vi "Búsqueda_Receta.vi"(10 "Receta":T2 {"Recetas LS Electric"."Modbus LS-Electric"."Delay respuesta" min=1 max=250 format="%.0f mseg."; "Recetas LS Electric"."Modbus LS-Electric"."Formato RS485" items=["RTU 8-N-1", "RTU 8-N-2", "RTU 8-E-1", "RTU 8-O-1"]; "Recetas LS Electric"."Modbus LS-Electric"."Velocidad datos" items=["1200 bps", "2400 bps", "4800 bps", "9600 bps", "19200 bps", "38400 bps", "56 kbps", "115 kbps"]; "Recetas LS Electric"."Modbus LS-Electric"."Identificador" min=1 max=250; "Recetas LS Electric"."Motor LS-Electric"."Voltaje nominal" min=170 max=480 format="%.0f V"; "Recetas LS Electric"."Motor LS-Electric"."Potencia nominal" items=["0.2 kW", "0.4 kW", "0.75 kW", "1.1 kW", "1.5 kW", "2.2 kW", "3.0 kW", "3.7 kW", "4.0 kW", "5.5 kW", "7.5 kW", "11.kW"]; "Recetas LS Electric"."Motor LS-Electric"."T. Desaceleración" format="%#_g seg"; "Recetas LS Electric"."Motor LS-Electric"."T. Aceleración" format="%#_g seg"; "Recetas LS Electric"."Motor LS-Electric"."Frecuencia máxima" format="%#_g Hz"; "Recetas LS Electric"."Motor LS-Electric"."Frecuencia mínima" format="%#_g Hz"; "Recetas LS Electric"."Motor LS-Electric"."Polos" min=2 max=48; "Recetas LS Electric"."Motor LS-Electric"."Velocidad nominal" format="%.0f rpm"; "Recetas LS Electric"."Motor LS-Electric"."Corriente nominal" format="%#_g Amp"; "Recetas LS Electric"."Motor LS-Electric"."Corriente sin carga" format="%#_g Amp"; "Recetas LS Electric"."Motor LS-Electric"."Frecuencia nominal" items=["60 Hz", "50 Hz"]; "Recetas LS Electric"."Referencias LS-Electric"."Referencia velocidad 2" items=["No asignar"=0, "Analógica (AI1)"=1, "Analógica (AI2)"=2, "Analógica (AI3)"=3, "Modbus"=164, "Potenciómetro (AIU1)"=183]; "Recetas LS Electric"."Referencias LS-Electric"."Referencia arranque 2" items=["Terminales"=1, "Modbus"=10]; "Recetas LS Electric"."Referencias LS-Electric"."Referencia velocidad 1" items=["No asignar"=0, "Analógica (AI1)"=1, "Analógica (AI2)"=2, "Analógica (AI3)"=3, "Modbus"=164, "Potenciómetro (AIU1)"=183]; "Recetas LS Electric"."Referencias LS-Electric"."Referencia arranque 1" items=["Terminales"=1, "Modbus"=10]; "Recetas LS Electric"."I/O LS-Electric"."Relevador 2" items=["Modbus"=0, "FDT-1"=1, "FDT-2"=2, "FDT-3"=3, "FDT-4"=4, "Sobrecarga"=5, "Sobrevoltaje"=10, "Bajo voltaje"=11, "Sobrecalentamiento"=12, "RUN"=14, "STOP"=15, "Listo"=22]; "Recetas LS Electric"."I/O LS-Electric"."Relevador 1" items=["Modbus"=0, "FDT-1"=1, "FDT-2"=2, "FDT-3"=3, "FDT-4"=4, "Sobrecarga"=5, "Sobrevoltaje"=10, "Bajo voltaje"=11, "Sobrecalentamiento"=12, "RUN"=14, "STOP"=15, "Listo"=22]; "Recetas LS Electric"."I/O LS-Electric"."Entrada 5 (P5)" items=["No asignar"=0, "FWD"=1, "REV"=2, "Reset"=3, "Fallo auxiliar (BX)"=5, "Habilitar RUN"=13, "3 hilos"=14, "Segunda referencia"=15, "Segundo motor"=26]; "Recetas LS Electric"."I/O LS-Electric"."Entrada 4 (P4)" items=["Sin asignar"=0, "FWD"=1, "REV"=2, "Reset"=3, "Fallo auxiliar (BX)"=5, "Habilitar RUN"=13, "3 hilos"=14, "Segunda referencia"=15, "Segundo motor"=26]; "Recetas LS Electric"."I/O LS-Electric"."Entrada 3 (P3)" items=["No asignar"=0, "FWD"=1, "REV"=2, "Reset"=3, "Fallo auxiliar (BX)"=5, "Habilitar RUN"=13, "3 hilos"=14, "Segunda referencia"=15, "Segundo motor"=26]; "Recetas LS Electric"."I/O LS-Electric"."Entrada 2 (P2)" items=["No asignar"=0, "FWD"=1, "REV"=2, "Reset"=3, "Fallo auxiliar (BX)"=5, "Habilitar RUN"=13, "3 hilos"=14, "Segunda referencia"=15, "Segundo motor"=26]; "Recetas LS Electric"."I/O LS-Electric"."Entrada 1 (P1)" items=["No asignar"=0, "FWD"=1, "REV"=2, "Reset"=3, "Fallo auxiliar (BX)"=5, "Habilitar RUN"=13, "3 hilos"=14, "Segunda referencia"=15, "Segundo motor"=26]; "Recetas ABB"."Referencias ABB"."Referencia velocidad 2" items=["No asignar"=0, "Analógica (AI1)"=1, "Analógica (AI2)"=2, "Analógica (AI3)"=3, "Modbus"=164, "Potenciómetro (AIU1)"=183]; "Recetas ABB"."Referencias ABB"."Referencia arranque 2" items=["Terminales"=1, "Modbus"=10]; "Recetas ABB"."Referencias ABB"."Referencia velocidad 1" items=["No asignar"=0, "Analógica (AI1)"=1, "Analógica (AI2)"=2, "Analógica (AI3)"=3, "Modbus"=164, "Potenciómetro (AIU1)"=183]; "Recetas ABB"."Referencias ABB"."Referencia arranque 1" items=["Terminales"=1, "Modbus"=10]; "Recetas ABB"."I/O ABB"."Entrada 4 (DI4)" items=["Sin asignar"=0, "Referencia vel. 2"=1, "Referencia vel. 3"=2, "Fallo auxiliar"=12, "Reset"=13, "Entrada lógica 1"=24, "Entrada lógica 2"=25]; "Recetas ABB"."I/O ABB"."Entrada 3 (DI3)" items=["No asignar"=0, "Referencia vel. 2"=1, "Referencia vel. 3"=2, "Fallo auxiliar"=12, "Reset"=13, "Entrada lógica 1"=24, "Entrada lógica 2"=25]; "Recetas ABB"."I/O ABB"."Entrada 2 (DI2)" items=["No asignar"=0, "Referencia vel. 2"=1, "Referencia vel. 3"=2, "Fallo auxiliar"=12, "Reset"=13, "Entrada lógica 1"=24, "Entrada lógica 2"=25, "REV 2 hilos"=50, "DIR 3 hilos"=51]; "Recetas ABB"."I/O ABB"."Entrada 1 (DI1)" items=["No asignar"=0, "Referencia vel. 2"=1, "Referencia vel. 3"=2, "Fallo auxiliar"=12, "Reset"=13, "Entrada lógica 1"=24, "Entrada lógica 2"=25, "FWD 2 hilos"=48, "RUN 3 hilos"=49]; "Recetas Delta"."Referencias Delta"."Referencia velocidad 2" items=["No asignar"=0, "Analógica (AI1)"=1, "Analógica (AI2)"=2, "Analógica (AI3)"=3, "Modbus"=164, "Potenciómetro (AIU1)"=183]; "Recetas Delta"."Referencias Delta"."Referencia arranque 2" items=["Terminales"=1, "Modbus"=10]; "Recetas Delta"."Referencias Delta"."Referencia velocidad 1" items=["No asignar"=0, "Analógica (AI1)"=1, "Analógica (AI2)"=2, "Analógica (AI3)"=3, "Modbus"=164, "Potenciómetro (AIU1)"=183]; "Recetas Delta"."Referencias Delta"."Referencia arranque 1" items=["Terminales"=1, "Modbus"=10]; "Recetas Delta"."I/O Delta"."Entrada 6 (MI6)" items=["Listo/Fallo"=0, "A frecuencia"=1, "Alimentación"=2, "Sobrefrecuencia"=6, "Sobrecorriente"=7, "Sobretensión"=8, "Modbus"=13]; "Recetas Delta"."I/O Delta"."Entrada 5 (MI5)" items=["Listo/Fallo"=0, "A frecuencia"=1, "Alimentación"=2, "Sobrefrecuencia"=6, "Sobrecorriente"=7, "Sobretensión"=8, "Modbus"=13]; "Recetas Delta"."I/O Delta"."Entrada 4 (MI4)" items=["Sin asignar"=0, "Referencia vel. 2"=1, "Referencia vel. 3"=2, "Fallo auxiliar"=12, "Reset"=13, "Entrada lógica 1"=24, "Entrada lógica 2"=25]; "Recetas Delta"."I/O Delta"."Entrada 3 (MI3)" items=["No asignar"=0, "Referencia vel. 2"=1, "Referencia vel. 3"=2, "Fallo auxiliar"=12, "Reset"=13, "Entrada lógica 1"=24, "Entrada lógica 2"=25]; "Recetas Delta"."I/O Delta"."Entrada 2 (MI2)" items=["No asignar"=0, "Referencia vel. 2"=1, "Referencia vel. 3"=2, "Fallo auxiliar"=12, "Reset"=13, "Entrada lógica 1"=24, "Entrada lógica 2"=25, "REV 2 hilos"=50, "DIR 3 hilos"=51]; "Recetas Delta"."I/O Delta"."Entrada 1 (MI1)" items=["No asignar"=0, "Referencia vel. 2"=1, "Referencia vel. 3"=2, "Fallo auxiliar"=12, "Reset"=13, "Entrada lógica 1"=24, "Entrada lógica 2"=25, "FWD 2 hilos"=48, "RUN 3 hilos"=49]; "Recetas Schneider"."I/O Schneider"."Transistor" items=["Listo/Fallo"=0, "A frecuencia"=1, "Alimentación"=2, "Sobrefrecuencia"=6, "Sobrecorriente"=7, "Sobretensión"=8, "Modbus"=13]; "Recetas Schneider"."I/O Schneider"."Relevador 2 (R2)" items=["Listo/Fallo"=0, "A frecuencia"=1, "Alimentación"=2, "Sobrefrecuencia"=6, "Sobrecorriente"=7, "Sobretensión"=8, "Modbus"=13]; "Recetas Schneider"."I/O Schneider"."Relevador 1 (R1)" items=["Listo/Fallo"=0, "A frecuencia"=1, "Alimentación"=2, "Sobrefrecuencia"=6, "Sobrecorriente"=7, "Sobretensión"=8, "Modbus"=13]; "Recetas Schneider"."I/O Schneider"."Entrada 6 (DI6)" items=["Listo/Fallo"=0, "A frecuencia"=1, "Alimentación"=2, "Sobrefrecuencia"=6, "Sobrecorriente"=7, "Sobretensión"=8, "Modbus"=13]; "Recetas Schneider"."I/O Schneider"."Entrada 5 (DI5)" items=["Listo/Fallo"=0, "A frecuencia"=1, "Alimentación"=2, "Sobrefrecuencia"=6, "Sobrecorriente"=7, "Sobretensión"=8, "Modbus"=13]; "Recetas Schneider"."I/O Schneider"."Entrada 4 (DI4)" items=["Sin asignar"=0, "Referencia vel. 2"=1, "Referencia vel. 3"=2, "Fallo auxiliar"=12, "Reset"=13, "Entrada lógica 1"=24, "Entrada lógica 2"=25]; "Recetas Schneider"."I/O Schneider"."Entrada 3 (DI3)" items=["No asignar"=0, "Referencia vel. 2"=1, "Referencia vel. 3"=2, "Fallo auxiliar"=12, "Reset"=13, "Entrada lógica 1"=24, "Entrada lógica 2"=25]; "Recetas Schneider"."I/O Schneider"."Entrada 2 (DI2)" items=["No asignar"=0, "Referencia vel. 2"=1, "Referencia vel. 3"=2, "Fallo auxiliar"=12, "Reset"=13, "Entrada lógica 1"=24, "Entrada lógica 2"=25, "REV 2 hilos"=50, "DIR 3 hilos"=51]; "Recetas Schneider"."I/O Schneider"."Entrada 1 (DI1)" items=["No asignar"=0, "Referencia vel. 2"=1, "Referencia vel. 3"=2, "Fallo auxiliar"=12, "Reset"=13, "Entrada lógica 1"=24, "Entrada lógica 2"=25, "FWD 2 hilos"=48, "RUN 3 hilos"=49]; "Recetas Schneider"."Referencias Schneider"."Referencia velocidad 2" items=["No asignar"=0, "Analógica (AI1)"=1, "Analógica (AI2)"=2, "Analógica (AI3)"=3, "Modbus"=164, "Potenciómetro (AIU1)"=183]; "Recetas Schneider"."Referencias Schneider"."Referencia arranque 2" items=["Terminales"=1, "Modbus"=10]; "Recetas Schneider"."Referencias Schneider"."Referencia velocidad 1" items=["No asignar"=0, "Analógica (AI1)"=1, "Analógica (AI2)"=2, "Analógica (AI3)"=3, "Modbus"=164, "Potenciómetro (AIU1)"=183]; "Recetas Schneider"."Referencias Schneider"."Referencia arranque 1" items=["Terminales"=1, "Modbus"=10]; "Recetas Allen Bradley"."Modbus PowerFlex"."Tmp. pérdida comun." min=0.0 max=60.0 format="%#_g seg."; "Recetas Allen Bradley"."Modbus PowerFlex"."Identificador" min=1 max=247; "Recetas Allen Bradley"."Modbus PowerFlex"."Formato RS485" items=["RTU 8-N-1", "RTU 8-E-1", "RTU 8-O-1", "RTU 8-N-2", "RTU 8-E-2", "RTU 8-O-2"]; "Recetas Allen Bradley"."Modbus PowerFlex"."Acc. pérdida comun." items=["Fallo", "Paro inercia", "Paro", "Nada"]; "Recetas Allen Bradley"."Modbus PowerFlex"."Velocidad datos" items=["9600 bps", "2400 bps", "4800 bps", "9600 bps", "19200 bps", "38400 bps"]; "Recetas Allen Bradley"."Motor PowerFlex"."T. Desaleceración" format="%#_g seg"; "Recetas Allen Bradley"."Motor PowerFlex"."T. Aceleración" format="%#_g seg"; "Recetas Allen Bradley"."Motor PowerFlex"."Velocidad nominal" format="%.0f rpm"; "Recetas Allen Bradley"."Motor PowerFlex"."Voltaje nominal" format="%.0f V"; "Recetas Allen Bradley"."Motor PowerFlex"."Frecuencia nominal" format="%.0f Hz"; "Recetas Allen Bradley"."Motor PowerFlex"."Corriente sobrecarga" format="%#_g Amp"; "Recetas Allen Bradley"."Motor PowerFlex"."Corriente nominal" format="%#_g Amp"; "Recetas Allen Bradley"."Motor PowerFlex"."Polos" min=2 max=40; "Recetas Allen Bradley"."I/O PowerFlex"."Relevador" items=["Listo/Fallo"=0, "A frecuencia"=1, "Alimentación"=2, "Sobrefrecuencia"=6, "Sobrecorriente"=7, "Sobretensión"=8, "Modbus"=13]; "Recetas Allen Bradley"."I/O PowerFlex"."Entrada 6 (06)" items=["No asignar"=0, "Referencia vel. 2"=1, "Referencia vel. 3"=2, "Fallo auxiliar"=12, "Reset"=13, "Entrada lógica 1"=24, "Entrada lógica 2"=25]; "Recetas Allen Bradley"."I/O PowerFlex"."Entrada 5 (05)" items=["No asignar"=0, "Referencia vel. 2"=1, "Referencia vel. 3"=2, "Fallo auxiliar"=12, "Reset"=13, "Entrada lógica 1"=24, "Entrada lógica 2"=25]; "Recetas Allen Bradley"."I/O PowerFlex"."Entrada 3 (03)" items=["No asignar"=0, "Referencia vel. 2"=1, "Referencia vel. 3"=2, "Fallo auxiliar"=12, "Reset"=13, "Entrada lógica 1"=24, "Entrada lógica 2"=25, "REV 2 hilos"=50, "DIR 3 hilos"=51]; "Recetas Allen Bradley"."I/O PowerFlex"."Entrada 2 (02)" items=["No asignar"=0, "Referencia vel. 2"=1, "Referencia vel. 3"=2, "Fallo auxiliar"=12, "Reset"=13, "Entrada lógica 1"=24, "Entrada lógica 2"=25, "FWD 2 hilos"=48, "RUN 3 hilos"=49]; "Recetas Allen Bradley"."Referencias PowerFlex"."Referencia velocidad 2" items=["Potenciómetro"=1, "Teclado"=2, "Modbus"=3, "Analógica (0-10V)"=5, "Analógica (4-20mA)"=6]; "Recetas Allen Bradley"."Referencias PowerFlex"."Referencia arranque 2" items=["Teclado"=1, "Terminales"=2, "Modbus"=3]; "Recetas Allen Bradley"."Referencias PowerFlex"."Referencia velocidad 1" items=["Potenciómetro"=1, "Teclado"=2, "Modbus"=3, "Analógica (0-10V)"=5, "Analógica (4-20mA)"=6]; "Recetas Allen Bradley"."Referencias PowerFlex"."Referencia arranque 1" items=["Teclado"=1, "Terminales"=2, "Modbus"=3]}, 11 "Índice":u32) -> (1 "Recetas Out":T1={"Receta Allen Bradley"={"Referencias PowerFlex"={"Referencia arranque 1"=0, "Referencia velocidad 1"=0, "Referencia arranque 2"=0, "Referencia velocidad 2"=0, "Descargar"=FALSE}, "I/O PowerFlex"={"Entrada 2 (02)"=0, "Entrada 3 (03)"=0, "Entrada 5 (05)"=0, "Entrada 6 (06)"=0, "Relevador"=0, "Descargar"=FALSE}, "Motor PowerFlex"={"Voltaje nominal"=0, "Frecuencia nominal"=0, "Corriente sobrecarga"=0.0, "Corriente nominal"=0.0, "Polos"=2, "Velocidad nominal"=0, "T. Aceleración"=0.0, "T. Desaleceración"=0.0, "Descargar"=FALSE}, "Modbus PowerFlex"={"Velocidad datos"=0, "Identificador"=1, "Acc. pérdida comun."=0, "Tmp. pérdida comun."=1.0, "Formato RS485"=0, "Descargar"=FALSE}, "Índice"=0}, "Receta Schneider"={"Referencias Schneider"={"Referencia arranque 1"=0, "Referencia velocidad 1"=0, "Referencia arranque 2"=0, "Referencia velocidad 2"=0, "Descargar"=FALSE}, "I/O Schneider"={"Entrada 1 (DI1)"=0, "Entrada 2 (DI2)"=0, "Entrada 3 (DI3)"=0, "Entrada 4 (DI4)"=0, "Entrada 5 (DI5)"=0, "Entrada 6 (DI6)"=0, "Relevador 1 (R1)"=0, "Relevador 2 (R2)"=0, "Transistor"=0, "Descargar"=FALSE}, "Índice"=0}, "Receta Delta"={"Referencias Delta"={"Referencia arranque 1"=0, "Referencia velocidad 1"=0, "Referencia arranque 2"=0, "Referencia velocidad 2"=0, "Descargar"=FALSE}, "I/O Delta"={"Entrada 1 (MI1)"=0, "Entrada 2 (MI2)"=0, "Entrada 3 (MI3)"=0, "Entrada 4 (MI4)"=0, "Entrada 5 (MI5)"=0, "Entrada 6 (MI6)"=0, "Descargar"=FALSE}, "Índice"=0}, "Receta ABB"={"Referencias ABB"={"Referencia arranque 1"=0, "Referencia velocidad 1"=0, "Referencia arranque 2"=0, "Referencia velocidad 2"=0, "Descargar"=FALSE}, "I/O ABB"={"Entrada 1 (DI1)"=0, "Entrada 2 (DI2)"=0, "Entrada 3 (DI3)"=0, "Entrada 4 (DI4)"=0, "Descargar"=FALSE}, "Índice"=0}, "Receta LS Electric"={"Referencias LS-Electric"={"Referencia arranque 1"=0, "Referencia velocidad 1"=0, "Referencia arranque 2"=0, "Referencia velocidad 2"=0, "Descargar"=FALSE}, "I/O LS-Electric"={"Entrada 1 (P1)"=0, "Entrada 2 (P2)"=0, "Entrada 3 (P3)"=0, "Entrada 4 (P4)"=0, "Entrada 5 (P5)"=0, "Relevador 1"=0, "Relevador 2"=0, "Descargar"=FALSE}, "Motor LS-Electric"={"Frecuencia nominal"=0, "Polos"=2, "Velocidad nominal"=0, "Corriente nominal"=0.0, "Corriente sin carga"=0.0, "Voltaje nominal"=170, "Potencia nominal"=0, "Frecuencia mínima"=0.0, "Frecuencia máxima"=0.0, "T. Aceleración"=0.0, "T. Desaceleración"=0.0, "Descargar"=FALSE}, "Modbus LS-Electric"={"Identificador"=1, "Velocidad datos"=0, "Formato RS485"=0, "Delay respuesta"=1, "Descargar"=FALSE}, "Índice"=0}} {"Receta LS Electric"."Modbus LS-Electric"."Delay respuesta" min=1 max=250 format="%.0f mseg."; "Receta LS Electric"."Modbus LS-Electric"."Formato RS485" items=["RTU 8-N-1", "RTU 8-N-2", "RTU 8-E-1", "RTU 8-O-1"]; "Receta LS Electric"."Modbus LS-Electric"."Velocidad datos" items=["1200 bps", "2400 bps", "4800 bps", "9600 bps", "19200 bps", "38400 bps", "56 kbps", "115 kbps"]; "Receta LS Electric"."Modbus LS-Electric"."Identificador" min=1 max=250; "Receta LS Electric"."Motor LS-Electric"."Voltaje nominal" min=170 max=480 format="%.0f V"; "Receta LS Electric"."Motor LS-Electric"."Potencia nominal" items=["0.2 kW", "0.4 kW", "0.75 kW", "1.1 kW", "1.5 kW", "2.2 kW", "3.0 kW", "3.7 kW", "4.0 kW", "5.5 kW", "7.5 kW", "11.kW"]; "Receta LS Electric"."Motor LS-Electric"."T. Desaceleración" format="%#_g seg"; "Receta LS Electric"."Motor LS-Electric"."T. Aceleración" format="%#_g seg"; "Receta LS Electric"."Motor LS-Electric"."Frecuencia máxima" format="%#_g Hz"; "Receta LS Electric"."Motor LS-Electric"."Frecuencia mínima" format="%#_g Hz"; "Receta LS Electric"."Motor LS-Electric"."Polos" min=2 max=48; "Receta LS Electric"."Motor LS-Electric"."Velocidad nominal" format="%.0f rpm"; "Receta LS Electric"."Motor LS-Electric"."Corriente nominal" format="%#_g Amp"; "Receta LS Electric"."Motor LS-Electric"."Corriente sin carga" format="%#_g Amp"; "Receta LS Electric"."Motor LS-Electric"."Frecuencia nominal" items=["60 Hz", "50 Hz"]; "Receta LS Electric"."Referencias LS-Electric"."Referencia velocidad 2" items=["No asignar"=0, "Analógica (AI1)"=1, "Analógica (AI2)"=2, "Analógica (AI3)"=3, "Modbus"=164, "Potenciómetro (AIU1)"=183]; "Receta LS Electric"."Referencias LS-Electric"."Referencia arranque 2" items=["Terminales"=1, "Modbus"=10]; "Receta LS Electric"."Referencias LS-Electric"."Referencia velocidad 1" items=["No asignar"=0, "Analógica (AI1)"=1, "Analógica (AI2)"=2, "Analógica (AI3)"=3, "Modbus"=164, "Potenciómetro (AIU1)"=183]; "Receta LS Electric"."Referencias LS-Electric"."Referencia arranque 1" items=["Terminales"=1, "Modbus"=10]; "Receta LS Electric"."I/O LS-Electric"."Relevador 2" items=["Modbus"=0, "FDT-1"=1, "FDT-2"=2, "FDT-3"=3, "FDT-4"=4, "Sobrecarga"=5, "Sobrevoltaje"=10, "Bajo voltaje"=11, "Sobrecalentamiento"=12, "RUN"=14, "STOP"=15, "Listo"=22]; "Receta LS Electric"."I/O LS-Electric"."Relevador 1" items=["Modbus"=0, "FDT-1"=1, "FDT-2"=2, "FDT-3"=3, "FDT-4"=4, "Sobrecarga"=5, "Sobrevoltaje"=10, "Bajo voltaje"=11, "Sobrecalentamiento"=12, "RUN"=14, "STOP"=15, "Listo"=22]; "Receta LS Electric"."I/O LS-Electric"."Entrada 5 (P5)" items=["No asignar"=0, "FWD"=1, "REV"=2, "Reset"=3, "Fallo auxiliar (BX)"=5, "Habilitar RUN"=13, "3 hilos"=14, "Segunda referencia"=15, "Segundo motor"=26]; "Receta LS Electric"."I/O LS-Electric"."Entrada 4 (P4)" items=["Sin asignar"=0, "FWD"=1, "REV"=2, "Reset"=3, "Fallo auxiliar (BX)"=5, "Habilitar RUN"=13, "3 hilos"=14, "Segunda referencia"=15, "Segundo motor"=26]; "Receta LS Electric"."I/O LS-Electric"."Entrada 3 (P3)" items=["No asignar"=0, "FWD"=1, "REV"=2, "Reset"=3, "Fallo auxiliar (BX)"=5, "Habilitar RUN"=13, "3 hilos"=14, "Segunda referencia"=15, "Segundo motor"=26]; "Receta LS Electric"."I/O LS-Electric"."Entrada 2 (P2)" items=["No asignar"=0, "FWD"=1, "REV"=2, "Reset"=3, "Fallo auxiliar (BX)"=5, "Habilitar RUN"=13, "3 hilos"=14, "Segunda referencia"=15, "Segundo motor"=26]; "Receta LS Electric"."I/O LS-Electric"."Entrada 1 (P1)" items=["No asignar"=0, "FWD"=1, "REV"=2, "Reset"=3, "Fallo auxiliar (BX)"=5, "Habilitar RUN"=13, "3 hilos"=14, "Segunda referencia"=15, "Segundo motor"=26]; "Receta ABB"."Referencias ABB"."Referencia velocidad 2" items=["No asignar"=0, "Analógica (AI1)"=1, "Analógica (AI2)"=2, "Analógica (AI3)"=3, "Modbus"=164, "Potenciómetro (AIU1)"=183]; "Receta ABB"."Referencias ABB"."Referencia arranque 2" items=["Terminales"=1, "Modbus"=10]; "Receta ABB"."Referencias ABB"."Referencia velocidad 1" items=["No asignar"=0, "Analógica (AI1)"=1, "Analógica (AI2)"=2, "Analógica (AI3)"=3, "Modbus"=164, "Potenciómetro (AIU1)"=183]; "Receta ABB"."Referencias ABB"."Referencia arranque 1" items=["Terminales"=1, "Modbus"=10]; "Receta ABB"."I/O ABB"."Entrada 4 (DI4)" items=["Sin asignar"=0, "Referencia vel. 2"=1, "Referencia vel. 3"=2, "Fallo auxiliar"=12, "Reset"=13, "Entrada lógica 1"=24, "Entrada lógica 2"=25]; "Receta ABB"."I/O ABB"."Entrada 3 (DI3)" items=["No asignar"=0, "Referencia vel. 2"=1, "Referencia vel. 3"=2, "Fallo auxiliar"=12, "Reset"=13, "Entrada lógica 1"=24, "Entrada lógica 2"=25]; "Receta ABB"."I/O ABB"."Entrada 2 (DI2)" items=["No asignar"=0, "Referencia vel. 2"=1, "Referencia vel. 3"=2, "Fallo auxiliar"=12, "Reset"=13, "Entrada lógica 1"=24, "Entrada lógica 2"=25, "REV 2 hilos"=50, "DIR 3 hilos"=51]; "Receta ABB"."I/O ABB"."Entrada 1 (DI1)" items=["No asignar"=0, "Referencia vel. 2"=1, "Referencia vel. 3"=2, "Fallo auxiliar"=12, "Reset"=13, "Entrada lógica 1"=24, "Entrada lógica 2"=25, "FWD 2 hilos"=48, "RUN 3 hilos"=49]; "Receta Delta"."Referencias Delta"."Referencia velocidad 2" items=["No asignar"=0, "Analógica (AI1)"=1, "Analógica (AI2)"=2, "Analógica (AI3)"=3, "Modbus"=164, "Potenciómetro (AIU1)"=183]; "Receta Delta"."Referencias Delta"."Referencia arranque 2" items=["Terminales"=1, "Modbus"=10]; "Receta Delta"."Referencias Delta"."Referencia velocidad 1" items=["No asignar"=0, "Analógica (AI1)"=1, "Analógica (AI2)"=2, "Analógica (AI3)"=3, "Modbus"=164, "Potenciómetro (AIU1)"=183]; "Receta Delta"."Referencias Delta"."Referencia arranque 1" items=["Terminales"=1, "Modbus"=10]; "Receta Delta"."I/O Delta"."Entrada 6 (MI6)" items=["Listo/Fallo"=0, "A frecuencia"=1, "Alimentación"=2, "Sobrefrecuencia"=6, "Sobrecorriente"=7, "Sobretensión"=8, "Modbus"=13]; "Receta Delta"."I/O Delta"."Entrada 5 (MI5)" items=["Listo/Fallo"=0, "A frecuencia"=1, "Alimentación"=2, "Sobrefrecuencia"=6, "Sobrecorriente"=7, "Sobretensión"=8, "Modbus"=13]; "Receta Delta"."I/O Delta"."Entrada 4 (MI4)" items=["Sin asignar"=0, "Referencia vel. 2"=1, "Referencia vel. 3"=2, "Fallo auxiliar"=12, "Reset"=13, "Entrada lógica 1"=24, "Entrada lógica 2"=25]; "Receta Delta"."I/O Delta"."Entrada 3 (MI3)" items=["No asignar"=0, "Referencia vel. 2"=1, "Referencia vel. 3"=2, "Fallo auxiliar"=12, "Reset"=13, "Entrada lógica 1"=24, "Entrada lógica 2"=25]; "Receta Delta"."I/O Delta"."Entrada 2 (MI2)" items=["No asignar"=0, "Referencia vel. 2"=1, "Referencia vel. 3"=2, "Fallo auxiliar"=12, "Reset"=13, "Entrada lógica 1"=24, "Entrada lógica 2"=25, "REV 2 hilos"=50, "DIR 3 hilos"=51]; "Receta Delta"."I/O Delta"."Entrada 1 (MI1)" items=["No asignar"=0, "Referencia vel. 2"=1, "Referencia vel. 3"=2, "Fallo auxiliar"=12, "Reset"=13, "Entrada lógica 1"=24, "Entrada lógica 2"=25, "FWD 2 hilos"=48, "RUN 3 hilos"=49]; "Receta Schneider"."I/O Schneider"."Transistor" items=["Listo/Fallo"=0, "A frecuencia"=1, "Alimentación"=2, "Sobrefrecuencia"=6, "Sobrecorriente"=7, "Sobretensión"=8, "Modbus"=13]; "Receta Schneider"."I/O Schneider"."Relevador 2 (R2)" items=["Listo/Fallo"=0, "A frecuencia"=1, "Alimentación"=2, "Sobrefrecuencia"=6, "Sobrecorriente"=7, "Sobretensión"=8, "Modbus"=13]; "Receta Schneider"."I/O Schneider"."Relevador 1 (R1)" items=["Listo/Fallo"=0, "A frecuencia"=1, "Alimentación"=2, "Sobrefrecuencia"=6, "Sobrecorriente"=7, "Sobretensión"=8, "Modbus"=13]; "Receta Schneider"."I/O Schneider"."Entrada 6 (DI6)" items=["Listo/Fallo"=0, "A frecuencia"=1, "Alimentación"=2, "Sobrefrecuencia"=6, "Sobrecorriente"=7, "Sobretensión"=8, "Modbus"=13]; "Receta Schneider"."I/O Schneider"."Entrada 5 (DI5)" items=["Listo/Fallo"=0, "A frecuencia"=1, "Alimentación"=2, "Sobrefrecuencia"=6, "Sobrecorriente"=7, "Sobretensión"=8, "Modbus"=13]; "Receta Schneider"."I/O Schneider"."Entrada 4 (DI4)" items=["Sin asignar"=0, "Referencia vel. 2"=1, "Referencia vel. 3"=2, "Fallo auxiliar"=12, "Reset"=13, "Entrada lógica 1"=24, "Entrada lógica 2"=25]; "Receta Schneider"."I/O Schneider"."Entrada 3 (DI3)" items=["No asignar"=0, "Referencia vel. 2"=1, "Referencia vel. 3"=2, "Fallo auxiliar"=12, "Reset"=13, "Entrada lógica 1"=24, "Entrada lógica 2"=25]; "Receta Schneider"."I/O Schneider"."Entrada 2 (DI2)" items=["No asignar"=0, "Referencia vel. 2"=1, "Referencia vel. 3"=2, "Fallo auxiliar"=12, "Reset"=13, "Entrada lógica 1"=24, "Entrada lógica 2"=25, "REV 2 hilos"=50, "DIR 3 hilos"=51]; "Receta Schneider"."I/O Schneider"."Entrada 1 (DI1)" items=["No asignar"=0, "Referencia vel. 2"=1, "Referencia vel. 3"=2, "Fallo auxiliar"=12, "Reset"=13, "Entrada lógica 1"=24, "Entrada lógica 2"=25, "FWD 2 hilos"=48, "RUN 3 hilos"=49]; "Receta Schneider"."Referencias Schneider"."Referencia velocidad 2" items=["No asignar"=0, "Analógica (AI1)"=1, "Analógica (AI2)"=2, "Analógica (AI3)"=3, "Modbus"=164, "Potenciómetro (AIU1)"=183]; "Receta Schneider"."Referencias Schneider"."Referencia arranque 2" items=["Terminales"=1, "Modbus"=10]; "Receta Schneider"."Referencias Schneider"."Referencia velocidad 1" items=["No asignar"=0, "Analógica (AI1)"=1, "Analógica (AI2)"=2, "Analógica (AI3)"=3, "Modbus"=164, "Potenciómetro (AIU1)"=183]; "Receta Schneider"."Referencias Schneider"."Referencia arranque 1" items=["Terminales"=1, "Modbus"=10]; "Receta Allen Bradley"."Modbus PowerFlex"."Tmp. pérdida comun." min=0.0 max=60.0 format="%#_g seg."; "Receta Allen Bradley"."Modbus PowerFlex"."Identificador" min=1 max=247; "Receta Allen Bradley"."Modbus PowerFlex"."Formato RS485" items=["RTU 8-N-1", "RTU 8-E-1", "RTU 8-O-1", "RTU 8-N-2", "RTU 8-E-2", "RTU 8-O-2"]; "Receta Allen Bradley"."Modbus PowerFlex"."Acc. pérdida comun." items=["Fallo", "Paro inercia", "Paro", "Nada"]; "Receta Allen Bradley"."Modbus PowerFlex"."Velocidad datos" items=["9600 bps", "2400 bps", "4800 bps", "9600 bps", "19200 bps", "38400 bps"]; "Receta Allen Bradley"."Motor PowerFlex"."T. Desaleceración" format="%#_g seg"; "Receta Allen Bradley"."Motor PowerFlex"."T. Aceleración" format="%#_g seg"; "Receta Allen Bradley"."Motor PowerFlex"."Velocidad nominal" format="%.0f rpm"; "Receta Allen Bradley"."Motor PowerFlex"."Voltaje nominal" format="%.0f V"; "Receta Allen Bradley"."Motor PowerFlex"."Frecuencia nominal" format="%.0f Hz"; "Receta Allen Bradley"."Motor PowerFlex"."Corriente sobrecarga" format="%#_g Amp"; "Receta Allen Bradley"."Motor PowerFlex"."Corriente nominal" format="%#_g Amp"; "Receta Allen Bradley"."Motor PowerFlex"."Polos" min=2 max=40; "Receta Allen Bradley"."I/O PowerFlex"."Relevador" items=["Listo/Fallo"=0, "A frecuencia"=1, "Alimentación"=2, "Sobrefrecuencia"=6, "Sobrecorriente"=7, "Sobretensión"=8, "Modbus"=13]; "Receta Allen Bradley"."I/O PowerFlex"."Entrada 6 (06)" items=["No asignar"=0, "Referencia vel. 2"=1, "Referencia vel. 3"=2, "Fallo auxiliar"=12, "Reset"=13, "Entrada lógica 1"=24, "Entrada lógica 2"=25]; "Receta Allen Bradley"."I/O PowerFlex"."Entrada 5 (05)" items=["No asignar"=0, "Referencia vel. 2"=1, "Referencia vel. 3"=2, "Fallo auxiliar"=12, "Reset"=13, "Entrada lógica 1"=24, "Entrada lógica 2"=25]; "Receta Allen Bradley"."I/O PowerFlex"."Entrada 3 (03)" items=["No asignar"=0, "Referencia vel. 2"=1, "Referencia vel. 3"=2, "Fallo auxiliar"=12, "Reset"=13, "Entrada lógica 1"=24, "Entrada lógica 2"=25, "REV 2 hilos"=50, "DIR 3 hilos"=51]; "Receta Allen Bradley"."I/O PowerFlex"."Entrada 2 (02)" items=["No asignar"=0, "Referencia vel. 2"=1, "Referencia vel. 3"=2, "Fallo auxiliar"=12, "Reset"=13, "Entrada lógica 1"=24, "Entrada lógica 2"=25, "FWD 2 hilos"=48, "RUN 3 hilos"=49]; "Receta Allen Bradley"."Referencias PowerFlex"."Referencia velocidad 2" items=["Potenciómetro"=1, "Teclado"=2, "Modbus"=3, "Analógica (0-10V)"=5, "Analógica (4-20mA)"=6]; "Receta Allen Bradley"."Referencias PowerFlex"."Referencia arranque 2" items=["Teclado"=1, "Terminales"=2, "Modbus"=3]; "Receta Allen Bradley"."Referencias PowerFlex"."Referencia velocidad 1" items=["Potenciómetro"=1, "Teclado"=2, "Modbus"=3, "Analógica (0-10V)"=5, "Analógica (4-20mA)"=6]; "Receta Allen Bradley"."Referencias PowerFlex"."Referencia arranque 1" items=["Teclado"=1, "Terminales"=2, "Modbus"=3]}, 3 "Fabricante":u32)   [LabVIEW 2013]
panel:
  out "Índice out":u32
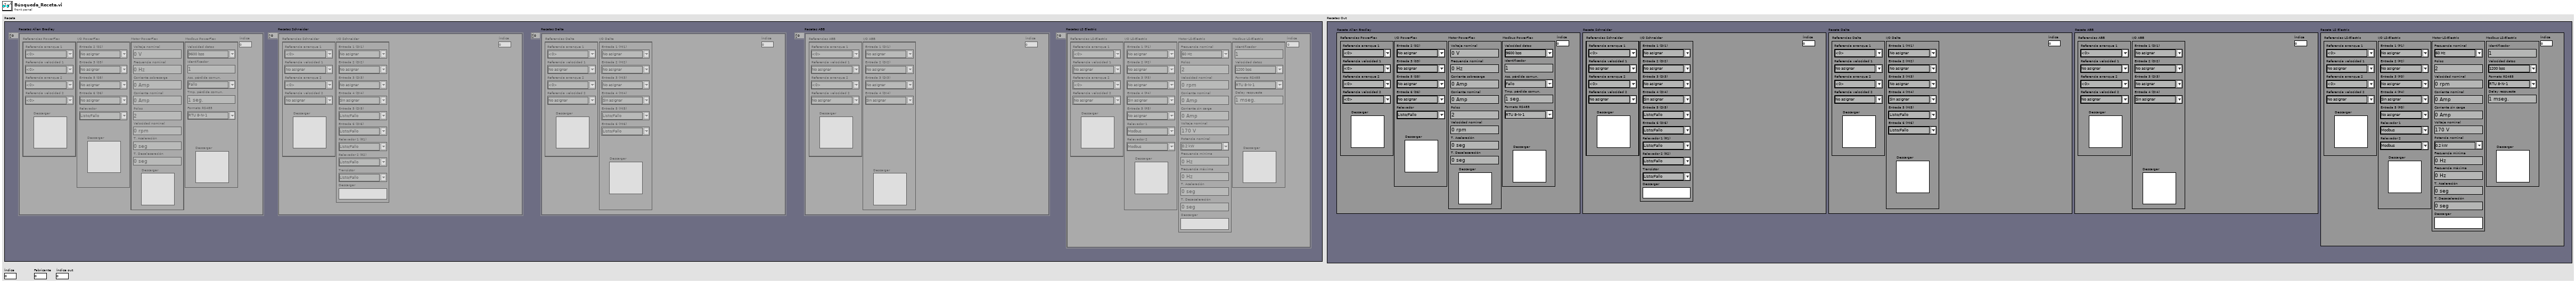
[diagram p1: front panel]
types:
  T1 = cluster{"Receta Allen Bradley":cluster{"Referencias PowerFlex":cluster{"Referencia arranque 1":u16, "Referencia velocidad 1":u16, "Referencia arranque 2":u16, "Referencia velocidad 2":u16, "Descargar":bool}, "I/O PowerFlex":cluster{"Entrada 2 (02)":u16, "Entrada 3 (03)":u16, "Entrada 5 (05)":u16, "Entrada 6 (06)":u16, "Relevador":u16, "Descargar":bool}, "Motor PowerFlex":cluster{"Voltaje nominal":u16, "Frecuencia nominal":u16, "Corriente sobrecarga":dbl, "Corriente nominal":dbl, "Polos":u16, "Velocidad nominal":u16, "T. Aceleración":dbl, "T. Desaleceración":dbl, "Descargar":bool}, "Modbus PowerFlex":cluster{"Velocidad datos":u16, "Identificador":u16, "Acc. pérdida comun.":u16, "Tmp. pérdida comun.":dbl, "Formato RS485":u16, "Descargar":bool}, "Índice":u32}, "Receta Schneider":cluster{"Referencias Schneider":cluster{"Referencia arranque 1":u16, "Referencia velocidad 1":u16, "Referencia arranque 2":u16, "Referencia velocidad 2":u16, "Descargar":bool}, "I/O Schneider":cluster{"Entrada 1 (DI1)":u16, "Entrada 2 (DI2)":u16, "Entrada 3 (DI3)":u16, "Entrada 4 (DI4)":u16, "Entrada 5 (DI5)":u16, "Entrada 6 (DI6)":u16, "Relevador 1 (R1)":u16, "Relevador 2 (R2)":u16, "Transistor":u16, "Descargar":bool}, "Índice":u32}, "Receta Delta":cluster{"Referencias Delta":cluster{"Referencia arranque 1":u16, "Referencia velocidad 1":u16, "Referencia arranque 2":u16, "Referencia velocidad 2":u16, "Descargar":bool}, "I/O Delta":cluster{"Entrada 1 (MI1)":u16, "Entrada 2 (MI2)":u16, "Entrada 3 (MI3)":u16, "Entrada 4 (MI4)":u16, "Entrada 5 (MI5)":u16, "Entrada 6 (MI6)":u16, "Descargar":bool}, "Índice":u32}, "Receta ABB":cluster{"Referencias ABB":cluster{"Referencia arranque 1":u16, "Referencia velocidad 1":u16, "Referencia arranque 2":u16, "Referencia velocidad 2":u16, "Descargar":bool}, "I/O ABB":cluster{"Entrada 1 (DI1)":u16, "Entrada 2 (DI2)":u16, "Entrada 3 (DI3)":u16, "Entrada 4 (DI4)":u16, "Descargar":bool}, "Índice":u32}, "Receta LS Electric":cluster{"Referencias LS-Electric":cluster{"Referencia arranque 1":u16, "Referencia velocidad 1":u16, "Referencia arranque 2":u16, "Referencia velocidad 2":u16, "Descargar":bool}, "I/O LS-Electric":cluster{"Entrada 1 (P1)":u16, "Entrada 2 (P2)":u16, "Entrada 3 (P3)":u16, "Entrada 4 (P4)":u16, "Entrada 5 (P5)":u16, "Relevador 1":u16, "Relevador 2":u16, "Descargar":bool}, "Motor LS-Electric":cluster{"Frecuencia nominal":u16, "Polos":u16, "Velocidad nominal":u16, "Corriente nominal":dbl, "Corriente sin carga":dbl, "Voltaje nominal":u16, "Potencia nominal":u16, "Frecuencia mínima":dbl, "Frecuencia máxima":dbl, "T. Aceleración":dbl, "T. Desaceleración":dbl, "Descargar":bool}, "Modbus LS-Electric":cluster{"Identificador":u16, "Velocidad datos":u16, "Formato RS485":u16, "Delay respuesta":u16, "Descargar":bool}, "Índice":u32}}
  T2 = cluster{"Recetas Allen Bradley":cluster{"Referencias PowerFlex":cluster{"Referencia arranque 1":u16, "Referencia velocidad 1":u16, "Referencia arranque 2":u16, "Referencia velocidad 2":u16, "Descargar":bool}, "I/O PowerFlex":cluster{"Entrada 2 (02)":u16, "Entrada 3 (03)":u16, "Entrada 5 (05)":u16, "Entrada 6 (06)":u16, "Relevador":u16, "Descargar":bool}, "Motor PowerFlex":cluster{"Voltaje nominal":u16, "Frecuencia nominal":u16, "Corriente sobrecarga":dbl, "Corriente nominal":dbl, "Polos":u16, "Velocidad nominal":u16, "T. Aceleración":dbl, "T. Desaleceración":dbl, "Descargar":bool}, "Modbus PowerFlex":cluster{"Velocidad datos":u16, "Identificador":u16, "Acc. pérdida comun.":u16, "Tmp. pérdida comun.":dbl, "Formato RS485":u16, "Descargar":bool}, "Índice":u32}[], "Recetas Schneider":cluster{"Referencias Schneider":cluster{"Referencia arranque 1":u16, "Referencia velocidad 1":u16, "Referencia arranque 2":u16, "Referencia velocidad 2":u16, "Descargar":bool}, "I/O Schneider":cluster{"Entrada 1 (DI1)":u16, "Entrada 2 (DI2)":u16, "Entrada 3 (DI3)":u16, "Entrada 4 (DI4)":u16, "Entrada 5 (DI5)":u16, "Entrada 6 (DI6)":u16, "Relevador 1 (R1)":u16, "Relevador 2 (R2)":u16, "Transistor":u16, "Descargar":bool}, "Índice":u32}[], "Recetas Delta":cluster{"Referencias Delta":cluster{"Referencia arranque 1":u16, "Referencia velocidad 1":u16, "Referencia arranque 2":u16, "Referencia velocidad 2":u16, "Descargar":bool}, "I/O Delta":cluster{"Entrada 1 (MI1)":u16, "Entrada 2 (MI2)":u16, "Entrada 3 (MI3)":u16, "Entrada 4 (MI4)":u16, "Entrada 5 (MI5)":u16, "Entrada 6 (MI6)":u16, "Descargar":bool}, "Índice":u32}[], "Recetas ABB":cluster{"Referencias ABB":cluster{"Referencia arranque 1":u16, "Referencia velocidad 1":u16, "Referencia arranque 2":u16, "Referencia velocidad 2":u16, "Descargar":bool}, "I/O ABB":cluster{"Entrada 1 (DI1)":u16, "Entrada 2 (DI2)":u16, "Entrada 3 (DI3)":u16, "Entrada 4 (DI4)":u16, "Descargar":bool}, "Índice":u32}[], "Recetas LS Electric":cluster{"Referencias LS-Electric":cluster{"Referencia arranque 1":u16, "Referencia velocidad 1":u16, "Referencia arranque 2":u16, "Referencia velocidad 2":u16, "Descargar":bool}, "I/O LS-Electric":cluster{"Entrada 1 (P1)":u16, "Entrada 2 (P2)":u16, "Entrada 3 (P3)":u16, "Entrada 4 (P4)":u16, "Entrada 5 (P5)":u16, "Relevador 1":u16, "Relevador 2":u16, "Descargar":bool}, "Motor LS-Electric":cluster{"Frecuencia nominal":u16, "Polos":u16, "Velocidad nominal":u16, "Corriente nominal":dbl, "Corriente sin carga":dbl, "Voltaje nominal":u16, "Potencia nominal":u16, "Frecuencia mínima":dbl, "Frecuencia máxima":dbl, "T. Aceleración":dbl, "T. Desaceleración":dbl, "Descargar":bool}, "Modbus LS-Electric":cluster{"Identificador":u16, "Velocidad datos":u16, "Formato RS485":u16, "Delay respuesta":u16, "Descargar":bool}, "Índice":u32}[]}
  T3 = cluster{"Referencias PowerFlex":cluster{"Referencia arranque 1":u16, "Referencia velocidad 1":u16, "Referencia arranque 2":u16, "Referencia velocidad 2":u16, "Descargar":bool}, "I/O PowerFlex":cluster{"Entrada 2 (02)":u16, "Entrada 3 (03)":u16, "Entrada 5 (05)":u16, "Entrada 6 (06)":u16, "Relevador":u16, "Descargar":bool}, "Motor PowerFlex":cluster{"Voltaje nominal":u16, "Frecuencia nominal":u16, "Corriente sobrecarga":dbl, "Corriente nominal":dbl, "Polos":u16, "Velocidad nominal":u16, "T. Aceleración":dbl, "T. Desaleceración":dbl, "Descargar":bool}, "Modbus PowerFlex":cluster{"Velocidad datos":u16, "Identificador":u16, "Acc. pérdida comun.":u16, "Tmp. pérdida comun.":dbl, "Formato RS485":u16, "Descargar":bool}, "Índice":u32}[]
  T4 = cluster{"Referencias Schneider":cluster{"Referencia arranque 1":u16, "Referencia velocidad 1":u16, "Referencia arranque 2":u16, "Referencia velocidad 2":u16, "Descargar":bool}, "I/O Schneider":cluster{"Entrada 1 (DI1)":u16, "Entrada 2 (DI2)":u16, "Entrada 3 (DI3)":u16, "Entrada 4 (DI4)":u16, "Entrada 5 (DI5)":u16, "Entrada 6 (DI6)":u16, "Relevador 1 (R1)":u16, "Relevador 2 (R2)":u16, "Transistor":u16, "Descargar":bool}, "Índice":u32}[]
  T5 = cluster{"Referencias Delta":cluster{"Referencia arranque 1":u16, "Referencia velocidad 1":u16, "Referencia arranque 2":u16, "Referencia velocidad 2":u16, "Descargar":bool}, "I/O Delta":cluster{"Entrada 1 (MI1)":u16, "Entrada 2 (MI2)":u16, "Entrada 3 (MI3)":u16, "Entrada 4 (MI4)":u16, "Entrada 5 (MI5)":u16, "Entrada 6 (MI6)":u16, "Descargar":bool}, "Índice":u32}[]
  T6 = cluster{"Referencias ABB":cluster{"Referencia arranque 1":u16, "Referencia velocidad 1":u16, "Referencia arranque 2":u16, "Referencia velocidad 2":u16, "Descargar":bool}, "I/O ABB":cluster{"Entrada 1 (DI1)":u16, "Entrada 2 (DI2)":u16, "Entrada 3 (DI3)":u16, "Entrada 4 (DI4)":u16, "Descargar":bool}, "Índice":u32}[]
  T7 = cluster{"Referencias LS-Electric":cluster{"Referencia arranque 1":u16, "Referencia velocidad 1":u16, "Referencia arranque 2":u16, "Referencia velocidad 2":u16, "Descargar":bool}, "I/O LS-Electric":cluster{"Entrada 1 (P1)":u16, "Entrada 2 (P2)":u16, "Entrada 3 (P3)":u16, "Entrada 4 (P4)":u16, "Entrada 5 (P5)":u16, "Relevador 1":u16, "Relevador 2":u16, "Descargar":bool}, "Motor LS-Electric":cluster{"Frecuencia nominal":u16, "Polos":u16, "Velocidad nominal":u16, "Corriente nominal":dbl, "Corriente sin carga":dbl, "Voltaje nominal":u16, "Potencia nominal":u16, "Frecuencia mínima":dbl, "Frecuencia máxima":dbl, "T. Aceleración":dbl, "T. Desaceleración":dbl, "Descargar":bool}, "Modbus LS-Electric":cluster{"Identificador":u16, "Velocidad datos":u16, "Formato RS485":u16, "Delay respuesta":u16, "Descargar":bool}, "Índice":u32}[]
  T8 = cluster{"Referencias PowerFlex":cluster{"Referencia arranque 1":u16, "Referencia velocidad 1":u16, "Referencia arranque 2":u16, "Referencia velocidad 2":u16, "Descargar":bool}, "I/O PowerFlex":cluster{"Entrada 2 (02)":u16, "Entrada 3 (03)":u16, "Entrada 5 (05)":u16, "Entrada 6 (06)":u16, "Relevador":u16, "Descargar":bool}, "Motor PowerFlex":cluster{"Voltaje nominal":u16, "Frecuencia nominal":u16, "Corriente sobrecarga":dbl, "Corriente nominal":dbl, "Polos":u16, "Velocidad nominal":u16, "T. Aceleración":dbl, "T. Desaleceración":dbl, "Descargar":bool}, "Modbus PowerFlex":cluster{"Velocidad datos":u16, "Identificador":u16, "Acc. pérdida comun.":u16, "Tmp. pérdida comun.":dbl, "Formato RS485":u16, "Descargar":bool}, "Índice":u32}
  T9 = cluster{"Referencias Schneider":cluster{"Referencia arranque 1":u16, "Referencia velocidad 1":u16, "Referencia arranque 2":u16, "Referencia velocidad 2":u16, "Descargar":bool}, "I/O Schneider":cluster{"Entrada 1 (DI1)":u16, "Entrada 2 (DI2)":u16, "Entrada 3 (DI3)":u16, "Entrada 4 (DI4)":u16, "Entrada 5 (DI5)":u16, "Entrada 6 (DI6)":u16, "Relevador 1 (R1)":u16, "Relevador 2 (R2)":u16, "Transistor":u16, "Descargar":bool}, "Índice":u32}
  T10 = cluster{"Referencias Delta":cluster{"Referencia arranque 1":u16, "Referencia velocidad 1":u16, "Referencia arranque 2":u16, "Referencia velocidad 2":u16, "Descargar":bool}, "I/O Delta":cluster{"Entrada 1 (MI1)":u16, "Entrada 2 (MI2)":u16, "Entrada 3 (MI3)":u16, "Entrada 4 (MI4)":u16, "Entrada 5 (MI5)":u16, "Entrada 6 (MI6)":u16, "Descargar":bool}, "Índice":u32}
  T11 = cluster{"Referencias ABB":cluster{"Referencia arranque 1":u16, "Referencia velocidad 1":u16, "Referencia arranque 2":u16, "Referencia velocidad 2":u16, "Descargar":bool}, "I/O ABB":cluster{"Entrada 1 (DI1)":u16, "Entrada 2 (DI2)":u16, "Entrada 3 (DI3)":u16, "Entrada 4 (DI4)":u16, "Descargar":bool}, "Índice":u32}
  T12 = cluster{"Referencias LS-Electric":cluster{"Referencia arranque 1":u16, "Referencia velocidad 1":u16, "Referencia arranque 2":u16, "Referencia velocidad 2":u16, "Descargar":bool}, "I/O LS-Electric":cluster{"Entrada 1 (P1)":u16, "Entrada 2 (P2)":u16, "Entrada 3 (P3)":u16, "Entrada 4 (P4)":u16, "Entrada 5 (P5)":u16, "Relevador 1":u16, "Relevador 2":u16, "Descargar":bool}, "Motor LS-Electric":cluster{"Frecuencia nominal":u16, "Polos":u16, "Velocidad nominal":u16, "Corriente nominal":dbl, "Corriente sin carga":dbl, "Voltaje nominal":u16, "Potencia nominal":u16, "Frecuencia mínima":dbl, "Frecuencia máxima":dbl, "T. Aceleración":dbl, "T. Desaceleración":dbl, "Descargar":bool}, "Modbus LS-Electric":cluster{"Identificador":u16, "Velocidad datos":u16, "Formato RS485":u16, "Delay respuesta":u16, "Descargar":bool}, "Índice":u32}
  T13 = cluster{"Recetas Allen Bradley":cluster{"Referencias PowerFlex":cluster{"Referencia arranque 1":u16, "Referencia velocidad 1":u16, "Referencia arranque 2":u16, "Referencia velocidad 2":u16, "Descargar":bool}, "I/O PowerFlex":cluster{"Entrada 2 (02)":u16, "Entrada 3 (03)":u16, "Entrada 5 (05)":u16, "Entrada 6 (06)":u16, "Relevador":u16, "Descargar":bool}, "Motor PowerFlex":cluster{"Voltaje nominal":u16, "Frecuencia nominal":u16, "Corriente sobrecarga":dbl, "Corriente nominal":dbl, "Polos":u16, "Velocidad nominal":u16, "T. Aceleración":dbl, "T. Desaleceración":dbl, "Descargar":bool}, "Modbus PowerFlex":cluster{"Velocidad datos":u16, "Identificador":u16, "Acc. pérdida comun.":u16, "Tmp. pérdida comun.":dbl, "Formato RS485":u16, "Descargar":bool}, "Índice":u32}, "Recetas Allen Bradley":cluster{"Referencias Schneider":cluster{"Referencia arranque 1":u16, "Referencia velocidad 1":u16, "Referencia arranque 2":u16, "Referencia velocidad 2":u16, "Descargar":bool}, "I/O Schneider":cluster{"Entrada 1 (DI1)":u16, "Entrada 2 (DI2)":u16, "Entrada 3 (DI3)":u16, "Entrada 4 (DI4)":u16, "Entrada 5 (DI5)":u16, "Entrada 6 (DI6)":u16, "Relevador 1 (R1)":u16, "Relevador 2 (R2)":u16, "Transistor":u16, "Descargar":bool}, "Índice":u32}, "Recetas Allen Bradley":cluster{"Referencias Delta":cluster{"Referencia arranque 1":u16, "Referencia velocidad 1":u16, "Referencia arranque 2":u16, "Referencia velocidad 2":u16, "Descargar":bool}, "I/O Delta":cluster{"Entrada 1 (MI1)":u16, "Entrada 2 (MI2)":u16, "Entrada 3 (MI3)":u16, "Entrada 4 (MI4)":u16, "Entrada 5 (MI5)":u16, "Entrada 6 (MI6)":u16, "Descargar":bool}, "Índice":u32}, "Recetas Allen Bradley":cluster{"Referencias ABB":cluster{"Referencia arranque 1":u16, "Referencia velocidad 1":u16, "Referencia arranque 2":u16, "Referencia velocidad 2":u16, "Descargar":bool}, "I/O ABB":cluster{"Entrada 1 (DI1)":u16, "Entrada 2 (DI2)":u16, "Entrada 3 (DI3)":u16, "Entrada 4 (DI4)":u16, "Descargar":bool}, "Índice":u32}, "Recetas Allen Bradley":cluster{"Referencias LS-Electric":cluster{"Referencia arranque 1":u16, "Referencia velocidad 1":u16, "Referencia arranque 2":u16, "Referencia velocidad 2":u16, "Descargar":bool}, "I/O LS-Electric":cluster{"Entrada 1 (P1)":u16, "Entrada 2 (P2)":u16, "Entrada 3 (P3)":u16, "Entrada 4 (P4)":u16, "Entrada 5 (P5)":u16, "Relevador 1":u16, "Relevador 2":u16, "Descargar":bool}, "Motor LS-Electric":cluster{"Frecuencia nominal":u16, "Polos":u16, "Velocidad nominal":u16, "Corriente nominal":dbl, "Corriente sin carga":dbl, "Voltaje nominal":u16, "Potencia nominal":u16, "Frecuencia mínima":dbl, "Frecuencia máxima":dbl, "T. Aceleración":dbl, "T. Desaceleración":dbl, "Descargar":bool}, "Modbus LS-Electric":cluster{"Identificador":u16, "Velocidad datos":u16, "Formato RS485":u16, "Delay respuesta":u16, "Descargar":bool}, "Índice":u32}}
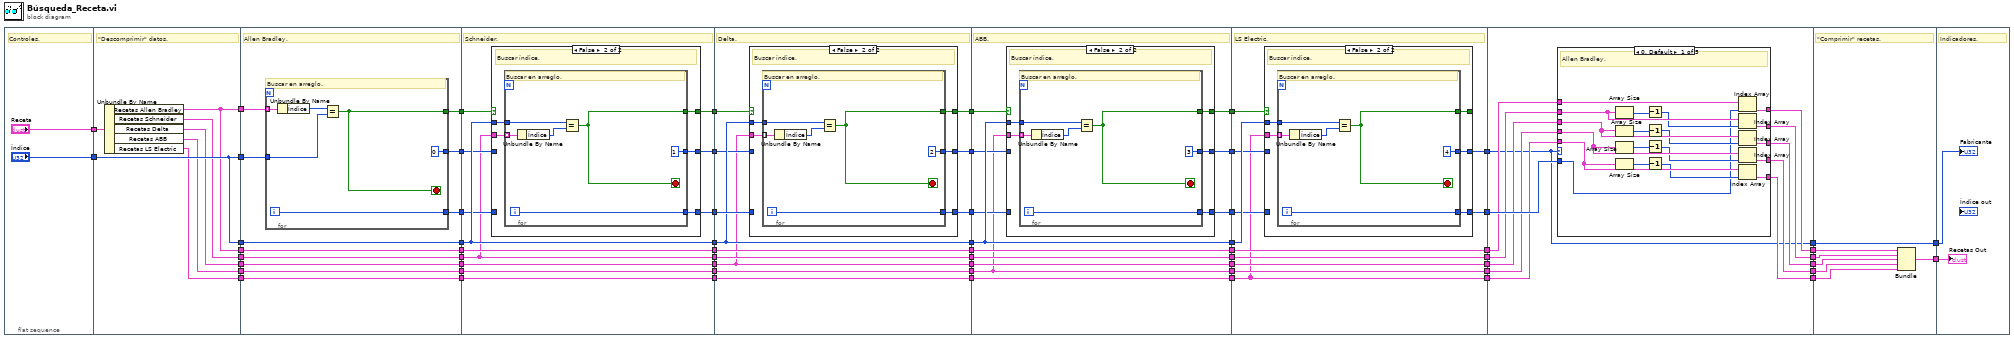
[diagram p0: block diagram]
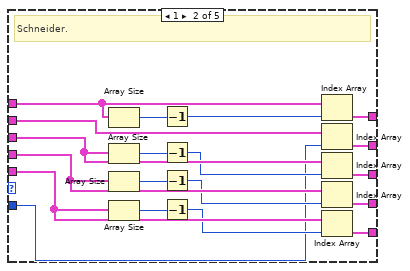
[diagram p6: hidden frame]
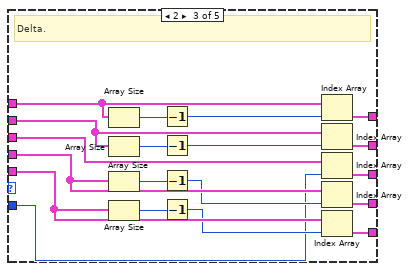
[diagram p7: hidden frame]
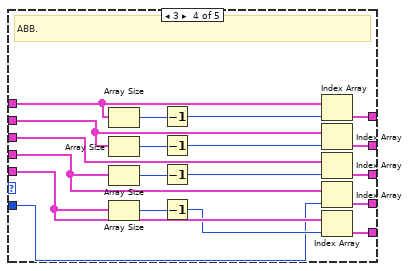
[diagram p8: hidden frame]
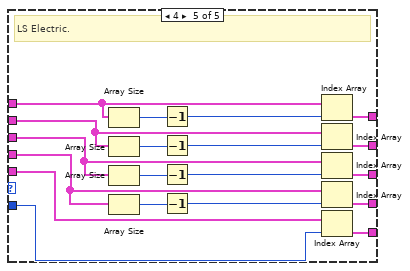
[diagram p9: hidden frame]
diagram:
  n1 = flat-sequence {
    tunnel: ["Receta"] -> w61
    tunnel: ["Índice"] -> w60
    tunnel: w61 -> [w69]
    tunnel: w60 -> [w70]
    tunnel: [w64] -> w59
    tunnel: [w70] -> w58
    tunnel: [w68] -> w57
    tunnel: [w67] -> w56
    tunnel: [w66] -> w55
    tunnel: [w65] -> w54
    tunnel: [w70] -> w26
    tunnel: [w64] -> w25
    tunnel: w59 -> [w81]
    tunnel: w58 -> [w73]
    tunnel: w57 -> [w80]
    tunnel: w56 -> [w79]
    tunnel: w55 -> [w78]
    tunnel: w54 -> [w77]
    tunnel: [w80] -> w53
    tunnel: [w79] -> w52
    tunnel: [w78] -> w51
    tunnel: [w77] -> w50
    tunnel: [w76] -> w49
    tunnel: [w72] -> w48
    tunnel: [w75] -> w47
    tunnel: [w74] -> w30
    tunnel: w26 -> [w72]
    tunnel: w25 -> [w71]
    tunnel: [w71] -> w24
    tunnel: w53 -> [w88]
    tunnel: w52 -> [w99]
    tunnel: w51 -> [w98]
    tunnel: w50 -> [w97]
    tunnel: w49 -> [w95]
    tunnel: w48 -> [w94]
    tunnel: w47 -> [w92]
    tunnel: [w99] -> w46
    tunnel: [w98] -> w45
    tunnel: [w97] -> w44
    tunnel: [w96] -> w43
    tunnel: [w94] -> w42
    tunnel: [w93] -> w41
    tunnel: w30 -> [w91]
    tunnel: [w90] -> w29
    tunnel: w24 -> [w89]
    tunnel: [w89] -> w23
    tunnel: [w88] -> w22
    tunnel: w46 -> [w114]
    tunnel: w45 -> [w125]
    tunnel: w44 -> [w124]
    tunnel: w43 -> [w123]
    tunnel: w42 -> [w119]
    tunnel: w41 -> [w122]
    tunnel: [w114] -> w40
    tunnel: [w125] -> w39
    tunnel: [w124] -> w38
    tunnel: [w121] -> w37
    tunnel: [w120] -> w36
    tunnel: [w119] -> w35
    tunnel: w29 -> [w118]
    tunnel: [w117] -> w28
    tunnel: w23 -> [w115]
    tunnel: w22 -> [w116]
    tunnel: [w116] -> w21
    tunnel: [w115] -> w20
    tunnel: w40 -> [w141]
    tunnel: w39 -> [w140]
    tunnel: w38 -> [w150]
    tunnel: w37 -> [w149]
    tunnel: w36 -> [w148]
    tunnel: w35 -> [w151]
    tunnel: [w150] -> w34
    tunnel: [w147] -> w33
    tunnel: [w146] -> w32
    tunnel: [w151] -> w31
    tunnel: w28 -> [w145]
    tunnel: [w144] -> w27
    tunnel: w21 -> [w142]
    tunnel: w20 -> [w143]
    tunnel: [w143] -> w19
    tunnel: [w142] -> w18
    tunnel: [w141] -> w17
    tunnel: [w140] -> w16
    tunnel: w34 -> [w166]
    tunnel: w33 -> [w176]
    tunnel: w32 -> [w174]
    tunnel: w31 -> [w175]
    tunnel: w27 -> [w172]
    tunnel: [w173] -> w15
    tunnel: [w171] -> w14
    tunnel: w19 -> [w169]
    tunnel: w18 -> [w168]
    tunnel: w17 -> [w167]
    tunnel: w16 -> [w170]
    tunnel: [w170] -> w13
    tunnel: [w169] -> w12
    tunnel: [w168] -> w11
    tunnel: [w167] -> w10
    tunnel: [w166] -> w9
    tunnel: w15 -> [w202]
    tunnel: w14 -> [w191]
    tunnel: w13 -> [w198]
    tunnel: [w193] -> w8
    tunnel: w12 -> [w201]
    tunnel: [w196] -> w7
    tunnel: w11 -> [w200]
    tunnel: [w195] -> w6
    tunnel: w10 -> [w199]
    tunnel: [w194] -> w5
    tunnel: w9 -> [w197]
    tunnel: [w192] -> w4
    tunnel: [w191] -> w2
    tunnel: w8 -> [w301]
    tunnel: w7 -> [w304]
    tunnel: w6 -> [w303]
    tunnel: w5 -> [w302]
    tunnel: w4 -> [w300]
    tunnel: [w299] -> w3
    tunnel: w2 -> [w298]
    tunnel: [w298] -> w1
    tunnel: w3 -> [w306]
    tunnel: w1 -> [w305]
    frame #0 {
      # "Controles."
    }
    frame #1 {
      # "\"Descomprimir\" datos."
      n2 = Unbundle By Name(w69) -> ("Recetas Allen Bradley"=w64:T3, "Recetas Schneider"=w68:T4, "Recetas Delta"=w67:T5, "Recetas ABB"=w66:T6, "Recetas LS Electric"=w65:T7)
    }
    frame #2 {
      # "Allen Bradley."
      n3 = for {
        tunnel: w81 -> [w87] mode=indexing
        tunnel: w73 -> [w85]
        tunnel: [w84] -> w76
        tunnel: [w83] -> w75
        tunnel: [0] -> w74
        i -> [w83]
        stop <- w84 stop-if-true
        # "Buscar en arreglo."
        n4 = Unbundle By Name(w87) -> ("Índice"=w86:u32)
        n5 = Equal?(x=w86, y=w85) -> (x = y?=w84:bool)
      }
    }
    frame #3 {
      # "Schneider."
      n6 = case shown="False" w95 {
        selector: w95 -> [w102 _]
        tunnel: w88 -> [_ w107]
        tunnel: w94 -> [_ w106]
        tunnel: [w102 w105] -> w96
        tunnel: w92 -> [w101 _]
        tunnel: [w101 w104] -> w93
        tunnel: w91 -> [w100 _]
        tunnel: [w100 w103] -> w90
        frame True {
          # "Nada."
        }
        frame False {
          # "Buscar índice."
          n7 = for {
            tunnel: w107 -> [w113] mode=indexing
            tunnel: w106 -> [w111]
            tunnel: [w112] -> w105
            tunnel: [w109] -> w104
            tunnel: [1] -> w103
            i -> [w109]
            stop <- w112 stop-if-true
            # "Buscar en arreglo."
            n8 = Unbundle By Name(w113) -> ("Índice"=w110:u32)
            n9 = Equal?(x=w111, y=w110) -> (x = y?=w112:bool)
          }
        }
      }
    }
    frame #4 {
      # "Delta."
      n10 = case shown="False" w123 {
        selector: w123 -> [w128 _]
        tunnel: w114 -> [_ w133]
        tunnel: w119 -> [_ w132]
        tunnel: [w128 w131] -> w121
        tunnel: w122 -> [w127 _]
        tunnel: [w127 w130] -> w120
        tunnel: w118 -> [w126 _]
        tunnel: [w126 w129] -> w117
        frame True {
          # "Nada."
        }
        frame False {
          # "Buscar índice."
          n11 = for {
            tunnel: w133 -> [w139] mode=indexing
            tunnel: w132 -> [w137]
            tunnel: [w138] -> w131
            tunnel: [w135] -> w130
            tunnel: [2] -> w129
            i -> [w135]
            stop <- w138 stop-if-true
            # "Buscar en arreglo."
            n12 = Unbundle By Name(w139) -> ("Índice"=w136:u32)
            n13 = Equal?(x=w137, y=w136) -> (x = y?=w138:bool)
          }
        }
      }
    }
    frame #5 {
      # "ABB."
      n14 = case shown="False" w149 {
        selector: w149 -> [w154 _]
        tunnel: w140 -> [_ w159]
        tunnel: w151 -> [_ w158]
        tunnel: [w154 w157] -> w147
        tunnel: w148 -> [w153 _]
        tunnel: [w153 w156] -> w146
        tunnel: w145 -> [w152 _]
        tunnel: [w152 w155] -> w144
        frame True {
          # "Nada."
        }
        frame False {
          # "Buscar índice."
          n15 = for {
            tunnel: w159 -> [w165] mode=indexing
            tunnel: w158 -> [w163]
            tunnel: [w164] -> w157
            tunnel: [w161] -> w156
            tunnel: [3] -> w155
            i -> [w161]
            stop <- w164 stop-if-true
            # "Buscar en arreglo."
            n16 = Unbundle By Name(w165) -> ("Índice"=w162:u32)
            n17 = Equal?(x=w163, y=w162) -> (x = y?=w164:bool)
          }
        }
      }
    }
    frame #6 {
      # "LS Electric."
      n18 = case shown="False" w176 {
        selector: w176 -> [w179 _]
        tunnel: w166 -> [_ w184]
        tunnel: w175 -> [_ w183]
        tunnel: [w179 w182] -> _
        tunnel: w174 -> [w178 _]
        tunnel: [w178 w181] -> w173
        tunnel: w172 -> [w177 _]
        tunnel: [w177 w180] -> w171
        frame True {
          # "Nada."
        }
        frame False {
          # "Buscar índice."
          n19 = for {
            tunnel: w184 -> [w190] mode=indexing
            tunnel: w183 -> [w188]
            tunnel: [w189] -> w182
            tunnel: [w186] -> w181
            tunnel: [4] -> w180
            i -> [w186]
            stop <- w189 stop-if-true
            # "Buscar en arreglo."
            n20 = Unbundle By Name(w190) -> ("Índice"=w187:u32)
            n21 = Equal?(x=w188, y=w187) -> (x = y?=w189:bool)
          }
        }
      }
    }
    frame #7 {
      n22 = case shown="0, Default" w191 {
        tunnel: w201 -> [w221 w223 w246 w266 w287]
        tunnel: w200 -> [w219 w239 w241 w262 w284]
        tunnel: w199 -> [w215 w236 w242 w263 w279]
        tunnel: w198 -> [w209 w230 w252 w271 w281]
        tunnel: w197 -> [w206 w227 w249 w269 w289]
        tunnel: w202 -> [w203 w224 w244 w261 w282]
        tunnel: [w220 w240 w259 w278 w297] -> w196
        tunnel: [w216 w237 w257 w276 w295] -> w195
        tunnel: [w214 w235 w256 w275 w294] -> w194
        tunnel: [w210 w231 w253 w272 w291] -> w193
        tunnel: [w204 w225 w247 w267 w288] -> w192
        frame 0, Default {
          # "Allen Bradley."
          n23 = Array Size(array=w219) -> (size(s)=w218:i32)
          n24 = Array Size(array=w215) -> (size(s)=w213:i32)
          n25 = Array Size(array=w209) -> (size(s)=w211:i32)
          n26 = Array Size(array=w206) -> (size(s)=w208:i32)
          n27 = Decrement(x=w218) -> (x-1=w217:i32)
          n28 = Decrement(x=w213) -> (x-1=w212:i32)
          n29 = Decrement(x=w211) -> (x-1=w207:i32)
          n30 = Decrement(x=w208) -> (x-1=w205:i32)
          n31 = Index Array(array=w221, index=w203) -> (element=w220:T8)
          n32 = Index Array(array=w219, index=w217) -> (element=w216:T9)
          n33 = Index Array(array=w215, index=w212) -> (element=w214:T10)
          n34 = Index Array(array=w209, index=w207) -> (element=w210:T11)
          n35 = Index Array(array=w206, index=w205) -> (element=w204:T12)
        }
        frame 1 {
          # "Schneider."
          n36 = Array Size(array=w223) -> (size(s)=w238:i32)
          n37 = Array Size(array=w236) -> (size(s)=w234:i32)
          n38 = Array Size(array=w230) -> (size(s)=w232:i32)
          n39 = Array Size(array=w227) -> (size(s)=w229:i32)
          n40 = Decrement(x=w238) -> (x-1=w222:i32)
          n41 = Decrement(x=w234) -> (x-1=w233:i32)
          n42 = Decrement(x=w232) -> (x-1=w228:i32)
          n43 = Decrement(x=w229) -> (x-1=w226:i32)
          n44 = Index Array(array=w223, index=w222) -> (element=w240:T8)
          n45 = Index Array(array=w239, index=w224) -> (element=w237:T9)
          n46 = Index Array(array=w236, index=w233) -> (element=w235:T10)
          n47 = Index Array(array=w230, index=w228) -> (element=w231:T11)
          n48 = Index Array(array=w227, index=w226) -> (element=w225:T12)
        }
        frame 2 {
          # "Delta."
          n49 = Array Size(array=w246) -> (size(s)=w258:i32)
          n50 = Array Size(array=w241) -> (size(s)=w255:i32)
          n51 = Array Size(array=w252) -> (size(s)=w254:i32)
          n52 = Array Size(array=w249) -> (size(s)=w251:i32)
          n53 = Decrement(x=w258) -> (x-1=w245:i32)
          n54 = Decrement(x=w255) -> (x-1=w243:i32)
          n55 = Decrement(x=w254) -> (x-1=w250:i32)
          n56 = Decrement(x=w251) -> (x-1=w248:i32)
          n57 = Index Array(array=w246, index=w245) -> (element=w259:T8)
          n58 = Index Array(array=w241, index=w243) -> (element=w257:T9)
          n59 = Index Array(array=w242, index=w244) -> (element=w256:T10)
          n60 = Index Array(array=w252, index=w250) -> (element=w253:T11)
          n61 = Index Array(array=w249, index=w248) -> (element=w247:T12)
        }
        frame 3 {
          # "ABB."
          n62 = Array Size(array=w266) -> (size(s)=w277:i32)
          n63 = Array Size(array=w262) -> (size(s)=w274:i32)
          n64 = Array Size(array=w271) -> (size(s)=w273:i32)
          n65 = Array Size(array=w269) -> (size(s)=w270:i32)
          n66 = Decrement(x=w277) -> (x-1=w265:i32)
          n67 = Decrement(x=w274) -> (x-1=w264:i32)
          n68 = Decrement(x=w273) -> (x-1=w260:i32)
          n69 = Decrement(x=w270) -> (x-1=w268:i32)
          n70 = Index Array(array=w266, index=w265) -> (element=w278:T8)
          n71 = Index Array(array=w262, index=w264) -> (element=w276:T9)
          n72 = Index Array(array=w263, index=w260) -> (element=w275:T10)
          n73 = Index Array(array=w271, index=w261) -> (element=w272:T11)
          n74 = Index Array(array=w269, index=w268) -> (element=w267:T12)
        }
        frame 4 {
          # "LS Electric."
          n75 = Array Size(array=w287) -> (size(s)=w296:i32)
          n76 = Array Size(array=w284) -> (size(s)=w293:i32)
          n77 = Array Size(array=w279) -> (size(s)=w292:i32)
          n78 = Array Size(array=w281) -> (size(s)=w290:i32)
          n79 = Decrement(x=w296) -> (x-1=w286:i32)
          n80 = Decrement(x=w293) -> (x-1=w285:i32)
          n81 = Decrement(x=w292) -> (x-1=w283:i32)
          n82 = Decrement(x=w290) -> (x-1=w280:i32)
          n83 = Index Array(array=w287, index=w286) -> (element=w297:T8)
          n84 = Index Array(array=w284, index=w285) -> (element=w295:T9)
          n85 = Index Array(array=w279, index=w283) -> (element=w294:T10)
          n86 = Index Array(array=w281, index=w280) -> (element=w291:T11)
          n87 = Index Array(array=w289, index=w282) -> (element=w288:T12)
        }
      }
    }
    frame #8 {
      # "\"Comprimir\" recetas."
      n88 = Bundle("Recetas Allen Bradley"=w304, "Recetas Allen Bradley"=w303, "Recetas Allen Bradley"=w302, "Recetas Allen Bradley"=w301, "Recetas Allen Bradley"=w300) -> (w299:T13)  [unwired: 1 in]
    }
    frame #9 {
      # "Indicadores."
      "Fabricante" <- w305
      "Recetas Out" <- w306
    }
  }
